vi "Create.vi"(8 "error in (no error)":errorcluster, 10 "Processes":set{string}(c389)) -> (0 "error out":errorcluster, 3 "Filter by Process out":refnum<class "Filter by Process.lvclass">)   [LabVIEW 2020, in "Filter by Process.lvclass"]
uses:
  Filter by Process.lvclass
  Filter by Process.lvclass/Filter by Process.ctl
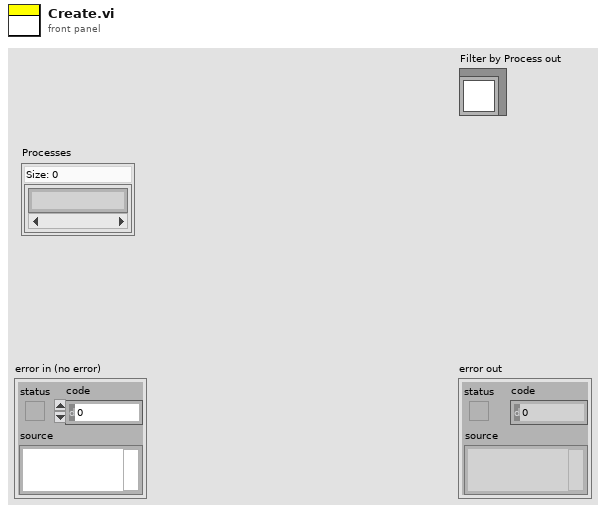
[diagram p1: front panel]
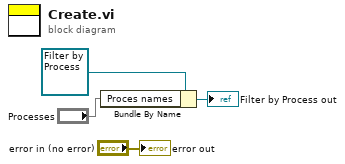
[diagram p0: block diagram]
diagram:
  n1 = Bundle By Name(cluster=refnum<class "Filter by Process.lvclass"> refnum ("Filter by Process out"), "Proces names"="Processes") -> (→"Filter by Process out":refnum<class "Filter by Process.lvclass">)
  "error out" <- "error in (no error)"
